vi "Prepare LV to Use Icon Editor Source v2.vi"(11 "Arguments":string[](array[string])) -> (2 "Output error":string, 3 "Exit code":i32)   [LabVIEW 2021]
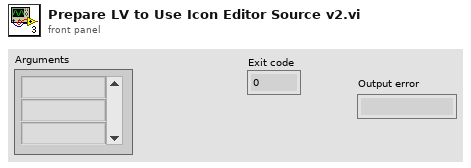
[diagram p1: front panel]
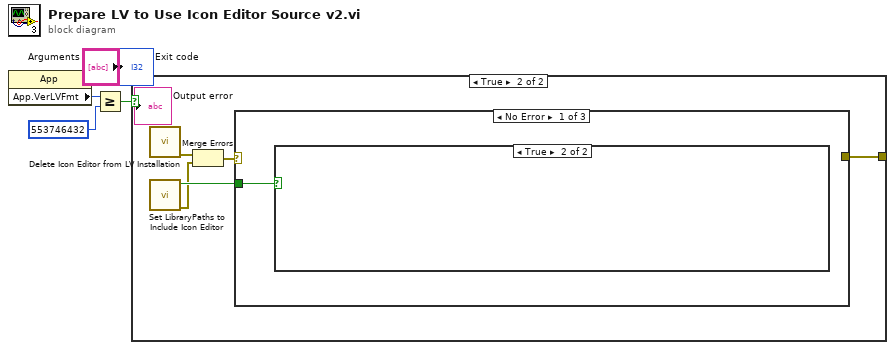
[diagram p0: block diagram]
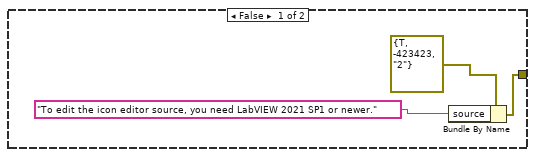
[diagram p2: hidden frame]
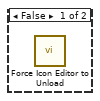
[diagram p3: hidden frame]
diagram:
  n1 = property class="App"() -> ("App.VerLVFmt"=w3:i32)  [unwired: 2 in, 2 out]
  n2 = Greater Or Equal?(x=w3, y=553746432 ("Application:Version As Integer")) -> (x >= y?=w1:bool)
  n3 = case shown="True" w1 {
    tunnel: [w5 w7] -> _
    frame False {
      n4 = Bundle By Name(cluster=errorcluster {"status"=TRUE, "code"=-423423, "source"="2"} ("error IO"), "source"="To edit the icon editor source, you need LabVIEW 2021 SP1 or newer." ("message")) -> (w5:errorcluster)
    }
    frame True {
      n5 = call "Delete Icon Editor from LV Installation.vi"() -> ("error out"=w10:errorcluster)  [unwired: 10 in, 1 out]
      n6 = call "Set LibraryPaths to Include Icon Editor.vi"() -> ("error out"=w8:errorcluster, "config modified?"=w11:bool)  [unwired: 10 in]
      n7 = Merge Errors(w10, w8) -> (w9:errorcluster)
      n8 = case shown="No Error" w9 {
        selector: w9 -> [_ w13 w14]
        tunnel: w11 -> [w12 _ _]
        tunnel: [_ w13 w14] -> w7
        frame No Error {
          n9 = case shown="True" w12 {
            frame False {
              n10 = call "Force Icon Editor to Unload.vi"() -> ()  [unwired: 12 in]
            }
            frame True {
            }
          }
        }
        frame Default {
        }
        frame Error {
          # "User cancelled, no further interaction needed"
        }
      }
    }
  }
